vi "Write Line UID.vi"(8 "error in (no error)":errorcluster, 10 "Line UID":string, 11 "Line in":refnum<class "Line.lvclass">) -> (0 "error out":errorcluster, 3 "Line out":refnum<class "Line.lvclass">)   [LabVIEW 2013, in "Table Manager.lvlib" / "Line.lvclass"]
uses:
  Line.lvclass
  Line.lvclass/Line.ctl
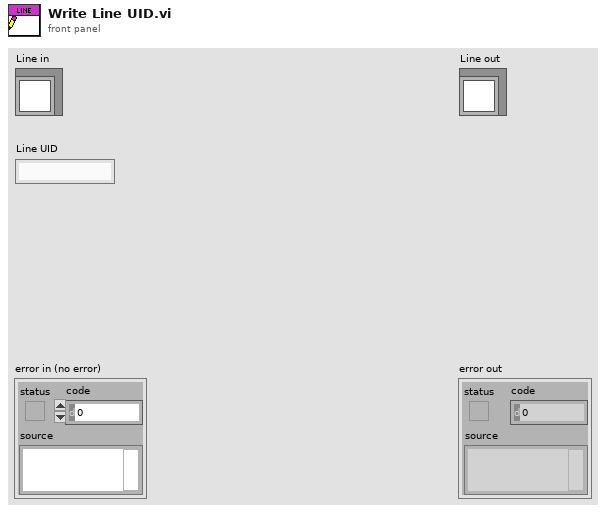
[diagram p1: front panel]
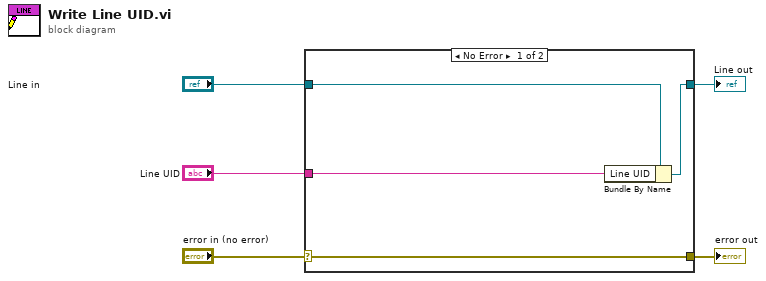
[diagram p0: block diagram]
diagram:
  n1 = case shown="No Error" "error in (no error)" {
    selector: "error in (no error)" -> [w9 w10]
    tunnel: [w9 w10] -> w4
    tunnel: [w7 w11] -> w2
    tunnel: "Line in" -> [w8 w11]
    tunnel: "Line UID" -> [w6 _]
    frame No Error {
      n2 = Bundle By Name(cluster=w8, "Line UID"=w6) -> (w7:refnum<class "Line.lvclass">)
    }
    frame Error {
    }
  }
  "error out" <- w4
  "Line out" <- w2
